vi "mxwScript_API_Option_TargetRef.vi"(4 "relativeToExistData":T1, 6 "terminalData":T2, 7 "targetRefType":T6, 8 "error in (no error)":errorcluster, 9 "templateData":T3={"tag"="", "index"=-1, "targetRefTemplateType"=enum."OutputAverage", "referencePosition"=enum."Right", "terminalData"={"name"="", "termIsTag"=FALSE, "referencePosition"=enum."TopLeft"}}, 10 "absoluteData":T5, 11 "options in":T7[](array[typedef])) -> (0 "error out":errorcluster, 3 "options out":T7[](array[typedef]))   [LabVIEW 2017]
doc: "Sets the default relationship between the template and block diagram reference points. This is used to calculate the drop position of templates."
uses:
  codeGenAPISupport.llb/cgAPI_mxwScript_OptionData.ctl
  codeGenAPISupport.llb/cgAPI_mxwScript_DrpTmplt_TargetRefType.ctl
  codeGenAPISupport.llb/cgAPI_mxwScript_DrpTmplt_AbsoluteData.ctl
  codeGenAPISupport.llb/cgAPI_mxwScript_DrpTmplt_TargetRefTemplateData.ctl
  codeGenAPISupport.llb/cgAPI_mxwScript_DrpTmplt_TargetRefTemplateType.ctl
  codeGenAPISupport.llb/cgAPI_mxwScript_DrpTmplt_ReferencePosition.ctl
  codeGenAPISupport.llb/cgAPI_mxwScript_DrpTmplt_TerminalData.ctl
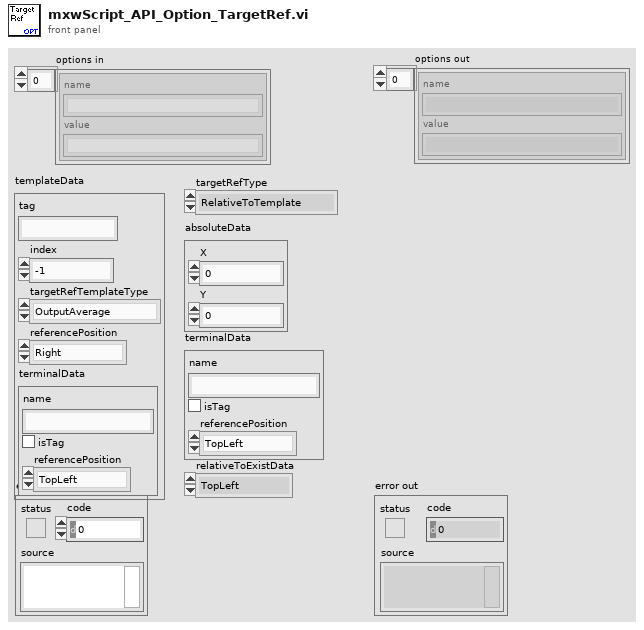
[diagram p1: front panel]
types:
  T1 = typedef "cgAPI_mxwScript_DrpTmplt_ReferencePosition.ctl" = enum16{"TopLeft", "Top", "TopRight", "Left", "Middle", "Right", "BottomLeft", "Bottom", "BottomRight"}
  T2 = typedef "cgAPI_mxwScript_DrpTmplt_TerminalData.ctl" = cluster{"name":string, "termIsTag":bool, "referencePosition":T1}
  T3 = typedef "cgAPI_mxwScript_DrpTmplt_TargetRefTemplateData.ctl" = cluster{"tag":string, "index":i32, "targetRefTemplateType":T4, "referencePosition":T1, "terminalData":T2}
  T4 = typedef "cgAPI_mxwScript_DrpTmplt_TargetRefTemplateType.ctl" = enum16{"OutputAverage", "Absolute", "Terminal"}
  T5 = typedef "cgAPI_mxwScript_DrpTmplt_AbsoluteData.ctl" = cluster{"X":i32, "Y":i32}
  T6 = typedef "cgAPI_mxwScript_DrpTmplt_TargetRefType.ctl" = enum16{"RelativeToTemplate", "RelativeToTerminal", "AbsoluteOnRoot", "AbsoluteOnTarget", "RelativeToExistOnRoot"}
  T7 = typedef "cgAPI_mxwScript_OptionData.ctl" = cluster{"name":string, "value":string}
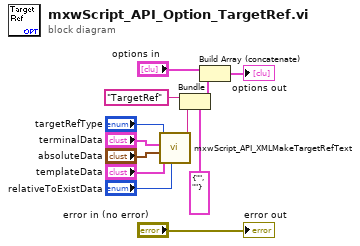
[diagram p0: block diagram]
diagram:
  n1 = call "mxwScript_API_XMLMakeTargetRefText.vi"("relativeToExistData"="relativeToExistData", "templateData"="templateData", "absoluteData"="absoluteData", "terminalData"="terminalData", "targetRefType"="targetRefType") -> ("targetRefText"=w3:string)  [unwired: 6 out]
  n2 = Bundle(cluster=T7 {"name"="", "value"=""} ("optionData"), "name"="TargetRef", "value"=w3) -> (w10:T7)
  n3 = Build Array (concatenate)("options in", w10) -> (→"options out":T7[])
  "error out" <- "error in (no error)"
